vi "IsArrayControl.vi"(8 "error in (no error)":errorcluster, 11 "Control reference in":refnum<vi>) -> (0 "error out":errorcluster, 2 "IsArrayControl":bool, 3 "Control reference out":refnum<vi>)   [LabVIEW 2020, in "MeasurementLink Measurement Server.lvlib"]
uses:
  MeasurementLink Measurement Server.lvlib
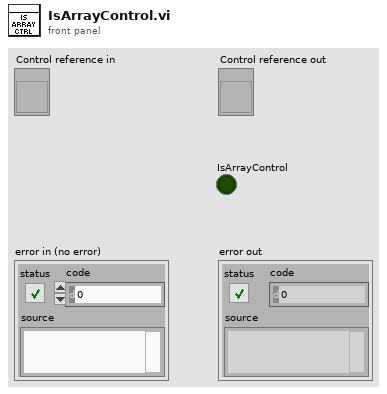
[diagram p1: front panel]
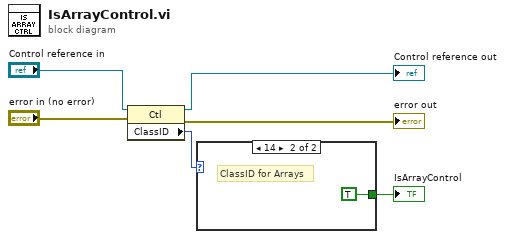
[diagram p0: block diagram]
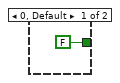
[diagram p2: hidden frame]
diagram:
  n1 = property class="Ctl"(reference="Control reference in", error in="error in (no error)") -> (reference out=→"Control reference out":refnum<vi>, error out=→"error out":errorcluster, "ClassID"=w6:u32)
  n2 = case shown="14" w6 {
    tunnel: [FALSE TRUE] -> w2
    frame 0, Default {
    }
    frame 14 {
      # "ClassID for Arrays"
    }
  }
  "IsArrayControl" <- w2
